vi "SetPropellerOutputPin.vi"(6 "error in (no error)":errorcluster, 8 "Pin Number":dbl, 9 "Value":bool, 10 "Dir":bool, 11 "SerialPortRef":T1) -> (0 "error out":errorcluster, 3 "SerialPortRef 2":T1)   [LabVIEW 2015]
uses:
  <vilib>/Rock Robotics/WPI/SerialPort/WPI_SerialPortRef.ctl
panel:
  out "Received":string
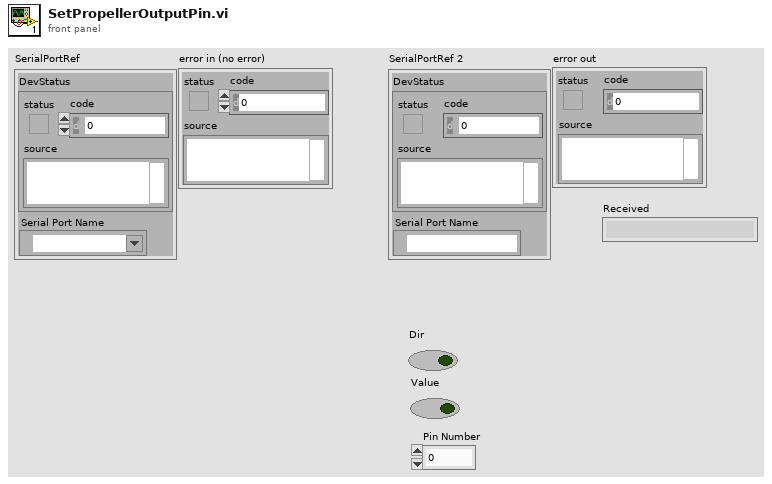
[diagram p1: front panel]
types:
  T1 = typedef "WPI_SerialPortRef.ctl" = cluster{"DevStatus":errorcluster, "Serial Port Name":refnum<visa-resource-name>}
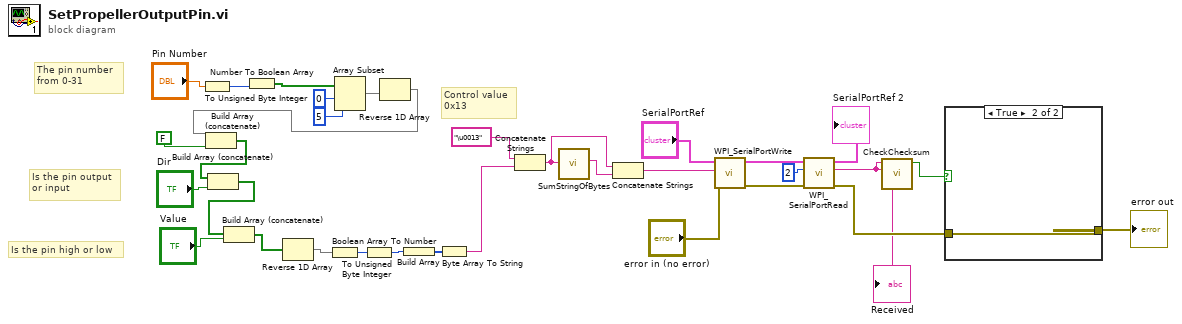
[diagram p0: block diagram]
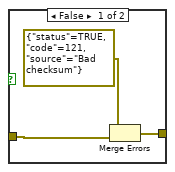
[diagram p2: hidden frame]
diagram:
  # "The pin number\nfrom 0-31"
  # "Is the pin high or low"
  # "Is the pin output\nor input"
  # "Control value\n0x13"
  n1 = To Unsigned Byte Integer(number="Pin Number") -> (unsigned 8bit integer=w25:u8)
  n2 = Number To Boolean Array(number=w25) -> (Boolean array=w18:bool[])
  n3 = Array Subset(array=w18, index=0, length=5) -> (w19:bool[])
  n4 = Reverse 1D Array(array=w19) -> (reversed array=w17:bool[])
  n5 = Build Array (concatenate)(w17, FALSE ("new element/subarray")) -> (w15:bool[])
  n6 = Build Array (concatenate)(w15, "Dir") -> (w12:bool[])
  n7 = Build Array (concatenate)(w12, "Value") -> (w11:bool[])
  n8 = Reverse 1D Array(array=w11) -> (reversed array=w10:bool[])
  n9 = Boolean Array To Number(Boolean array=w10) -> (number=w24:u32)
  n10 = To Unsigned Byte Integer(number=w24) -> (unsigned 8bit integer=w23:u8)
  n11 = Build Array(w23) -> (w22:u8[])
  n12 = Byte Array To String(unsigned byte array=w22) -> (string=w8:string)
  n13 = Concatenate Strings("\u0013" ("Buffer"), w8) -> (w6:string)
  n14 = call "SumStringOfBytes.vi"("String Of Bytes"=w6) -> ("SumAsString"=w7:string)  [unwired: 10 in]
  n15 = Concatenate Strings(w6, w7) -> (w5:string)
  n16 = call <vilib>:"WPI_SerialPortWrite.vi"("error in (no error)"="error in (no error)", "Buffer"=w5, "SerialPortRef"="SerialPortRef") -> ("error out"=w29:errorcluster, "SerialPortRef"=w30:T1)  [unwired: 6 in, 1 out]
  n17 = call <vilib>:"WPI_SerialPortRead.vi"("error in (no error)"=w29, "Num Bytes to Read"=u32 2, "SerialPortRef"=w30) -> ("error out"=w4:errorcluster, "Buffer"=w2:string, "SerialPortRef"=→"SerialPortRef 2":T1)  [unwired: 6 in]
  "Received" <- w2
  n18 = call "CheckChecksum.vi"("String"=w2) -> ("x = y?"=w1:bool)  [unwired: 10 in]
  n19 = case shown="True" w1 {
    tunnel: w4 -> [w34 w36]
    tunnel: [w33 w36] -> w3
    frame False {
      n20 = Merge Errors(errorcluster {"status"=TRUE, "code"=121, "source"="Bad checksum"} ("error in"), w34) -> (w33:errorcluster)
    }
    frame True {
    }
  }
  "error out" <- w3
